vi "Actor Event Wrapper.vi"(8 "Queue Mailbox":refnum<data-value>, 9 "Self Event Alias":string, 10 "Queue of Self Event":refnum<queue>, 11 "Event jettl":refnum<class "Event.lvclass">) -> ()   [LabVIEW 2021, in "jettl.lvlib" / "Base Event.lvlib"]
uses:
  Base Event.lvlib
  Event/Event.lvclass
  Msg Strategy/Msg Strategy.lvclass
  Addresses/Addresses/Addresses.lvclass
  Base Event/Base Event.lvclass
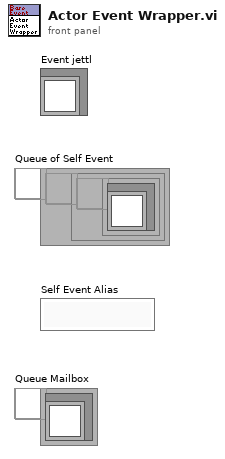
[diagram p1: front panel]
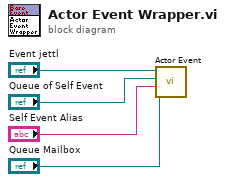
[diagram p0: block diagram]
diagram:
  n1 = call "Actor Event.vi"("Queue Mailbox"="Queue Mailbox", "Self Event Alias"="Self Event Alias", "Queue of Self Event"="Queue of Self Event", "Event"="Event jettl") -> ()  [unwired: 8 in]
